vi "Read Roles.vi"(8 "error in (no error)":errorcluster, 11 "PrepareKickoffAllyPlay in":refnum<class "PrepareKickoffAllyPlay.lvclass">) -> (0 "error out":errorcluster, 2 "Roles":T1, 3 "PrepareKickoffAllyPlay out":refnum<class "PrepareKickoffAllyPlay.lvclass">)   [LabVIEW 2023, in "PrepareKickoffAllyPlay.lvclass"]
uses:
  PrepareKickoffAllyPlay.lvclass
  AttackerAimGoalRole_class/AttackerAimGoalRole.lvclass
  FollowAttackerRole_class/FollowAttackerRole.lvclass
  PrepareKickoffAllyPlay.lvclass/PrepareKickoffAllyPlay.ctl
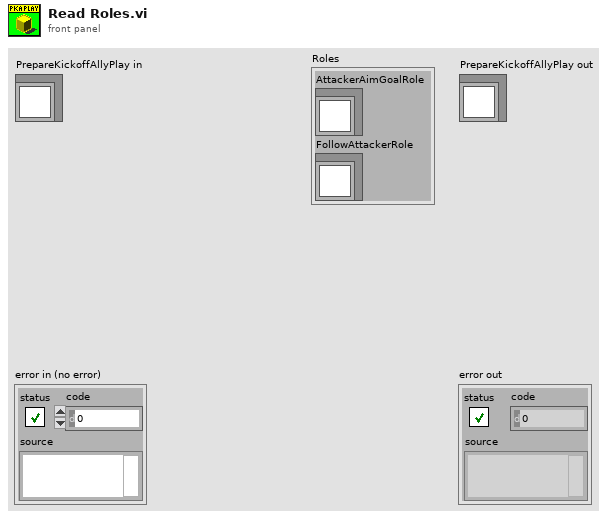
[diagram p1: front panel]
types:
  T1 = cluster{"AttackerAimGoalRole":refnum<class "AttackerAimGoalRole.lvclass">, "FollowAttackerRole":refnum<class "FollowAttackerRole.lvclass">}
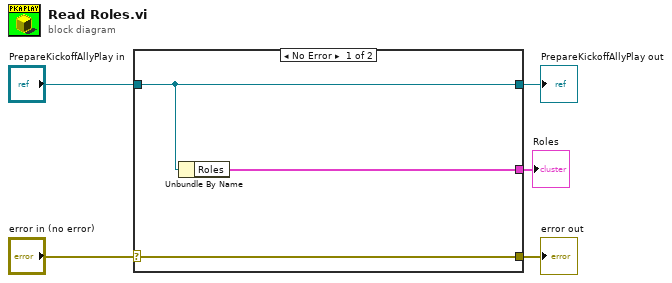
[diagram p0: block diagram]
diagram:
  n1 = case shown="No Error" "error in (no error)" {
    selector: "error in (no error)" -> [w8 w9]
    tunnel: [w8 w9] -> w4
    tunnel: [w7 w10] -> w2
    tunnel: "PrepareKickoffAllyPlay in" -> [w7 w10]
    tunnel: [w6 _] -> w1
    frame No Error {
      n2 = Unbundle By Name(w7) -> ("Roles"=w6:T1)
    }
    frame Error {
    }
  }
  "error out" <- w4
  "PrepareKickoffAllyPlay out" <- w2
  "Roles" <- w1
